vi "Add Timestamped Data.vi"(8 "Error In":errorcluster, 10 "X-t Value Pairs":cluster{"Time Stamp":timestamp, "Value":dbl}[](array[cluster]) {"Time Stamp" format="%<%x %.3X>T"}, 11 "BNT_XtGraph in":refnum<class "BNT_XtGraph.lvclass">) -> (0 "Error Out":errorcluster, 3 "BNT_XtGraph out":refnum<class "BNT_XtGraph.lvclass">)   [LabVIEW 2019, in "BNT_XtGraph.lvlib" / "BNT_XtGraph.lvclass"]
doc: "Add actual timestamped data to history."
uses:
  BNT_XtGraph.lvclass
  BNT_XtGraph.lvclass/BNT_XtGraph.ctl
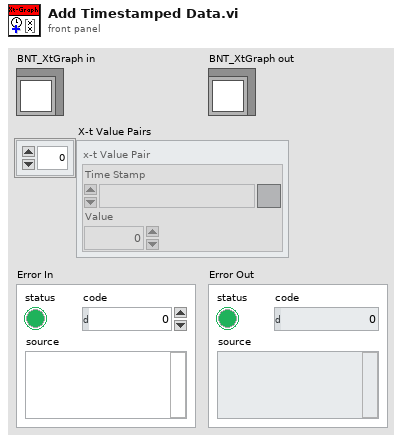
[diagram p1: front panel]
types:
  T1 = cluster{"X-t Value Pairs":cluster{"Time Stamp":timestamp, "Value":dbl}[]}[]
  T2 = cluster{"X-t Value Pairs":cluster{"Time Stamp":timestamp, "Value":dbl}[]}
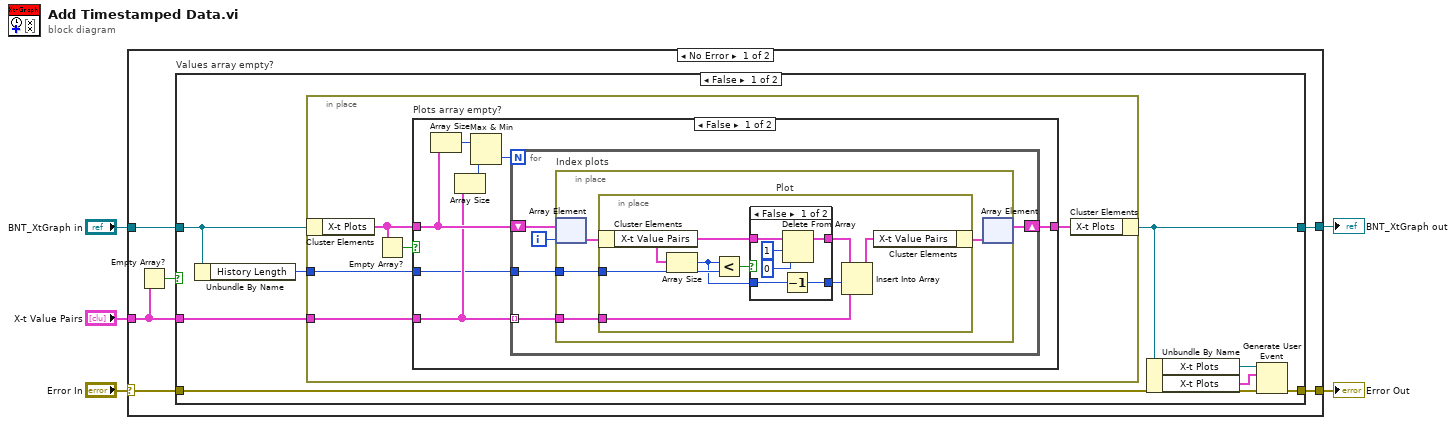
[diagram p0: block diagram]
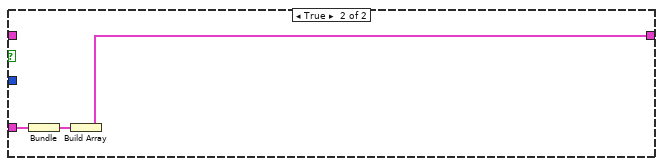
[diagram p3: hidden frame]
diagram:
  n1 = case shown="No Error" "Error In" {
    selector: "Error In" -> [w8 w63]
    tunnel: [w9 w63] -> w2
    tunnel: [w10 w62] -> w4
    tunnel: "BNT_XtGraph in" -> [w11 w62]
    tunnel: "X-t Value Pairs" -> [w6 _]
    frame No Error {
      n2 = Empty Array?(array=w6) -> (empty?=w7:bool)
      n3 = case "Values array empty?" shown="False" w7 {
        tunnel: w11 -> [w18 w61]
        tunnel: [w16 w61] -> w10
        tunnel: [w12 w60] -> w9
        tunnel: w8 -> [w13 w60]
        tunnel: w6 -> [w19 _]
        frame False {
          n4 = Unbundle By Name(w18) -> ("History Length"=w17:u32)
          n5 = in-place {
            in-place-border: w19 -> [w23]
            in-place-border: w17 -> [w20]
            n6 = in-place-cluster #1(w18) -> ("X-t Plots"=w21:T1)
            n7 = Empty Array?(array=w21) -> (empty?=w24:bool)
            n8 = case "Plots array empty?" shown="False" w24 {
              tunnel: w23 -> [w26 w57]
              tunnel: [w27 w59] -> w22
              tunnel: w21 -> [w28 _]
              tunnel: w20 -> [w25 _]
              frame False {
                n9 = Array Size(array=w28) -> (size(s)=w31:i32)
                n10 = Array Size(array=w26) -> (size(s)=w30:i32)
                n11 = Max & Min(x=w31, y=w30) -> (min(x,y)=w29:i32)  [unwired: 1 out]
                n12 = for {
                  N: w29 -> [_]
                  shift-right: [w34] -> w27
                  shift-left: w28 -> [w36]
                  tunnel: w26 -> [w33] mode=indexing
                  tunnel: w25 -> [w32]
                  i -> [w35]
                  n13 = in-place "Index plots" {
                    in-place-border: w33 -> [w38]
                    in-place-border: w32 -> [w37]
                    n14 = in-place-array #2(w36, w35) -> (w40:T2)
                    n15 = in-place "Plot" {
                      in-place-border: w38 -> [w41]
                      in-place-border: w37 -> [w46]
                      n16 = in-place-cluster #3(w40) -> ("X-t Value Pairs"=w47:cluster{"Time Stamp":timestamp, "Value":dbl}[])
                      n17 = Array Size(array=w47) -> (size(s)=w43:i32)
                      n18 = Less?(x=w43, y=w46) -> (x < y?=w48:bool)
                      n19 = case shown="False" w48 {
                        tunnel: w47 -> [w54 w56]
                        tunnel: [w53 w56] -> w45
                        tunnel: [w49 w55] -> w42
                        tunnel: w43 -> [w50 w55]
                        frame False {
                          n20 = Decrement(x=w50) -> (x-1=w49:i32)
                          n21 = Delete From Array(array=w54, length=1, index=0) -> (array with subset deleted=w53:cluster{"Time Stamp":timestamp, "Value":dbl}[])  [unwired: 1 out]
                        }
                        frame True {
                        }
                      }
                      n22 = Insert Into Array(array=w45, index=w42, new element=w41) -> (w44:cluster{"Time Stamp":timestamp, "Value":dbl}[])
                      n23 = in-place-cluster #3("X-t Value Pairs"=w44) -> (w39:T2)
                    }
                    n24 = in-place-array #2(w39) -> (w34:T1)  [unwired: 1 out]
                  }
                }
              }
              frame True {
                n25 = Bundle("X-t Value Pairs"=w57) -> (w58:T2)  [unwired: 1 in]
                n26 = Build Array(w58) -> (w59:T1)
              }
            }
            n27 = in-place-cluster #1("X-t Plots"=w22) -> (w16:refnum<class "BNT_XtGraph.lvclass">)
          }
          n28 = Unbundle By Name(w16) -> ("X-t Plots"=w15:refnum<user-event>, "X-t Plots"=w14:T1)
          n29 = Generate User Event(user event=w15, event data cluster=w14, error in=w13) -> (error out=w12:errorcluster)  [unwired: 1 in, 1 out]
        }
        frame True {
        }
      }
    }
    frame Error {
    }
  }
  "BNT_XtGraph out" <- w4
  "Error Out" <- w2
